vi "Listbox-Get Checked Items (1D Boolean).vi"(8 "error in (no error)":errorcluster, 11 "reference":refnum<vi>) -> (0 "error out":errorcluster, 3 "checked?":bool[](array[boolean]))   [LabVIEW 2015]
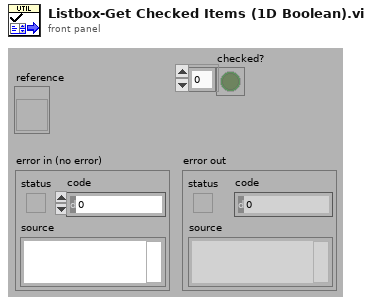
[diagram p1: front panel]
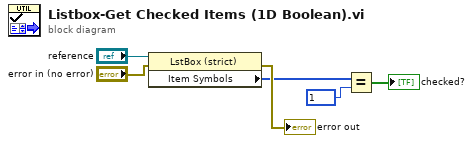
[diagram p0: block diagram]
diagram:
  n1 = property on="Property Node" class="LstBox (strict)"(reference="reference", error in="error in (no error)") -> (error out=→"error out":errorcluster, "Item Symbols"=w2:i32[])  [unwired: 1 out]
  n2 = Equal?(x=w2, y=1) -> (x = y?=→"checked?":bool[])
